vi "Main.vi"() -> ()   [LabVIEW 2014, in "SLL Tools Launcher.lvlib"]
uses:
  SLL Tools Launcher.lvlib
  Typedefs/SLL Tool.ctl
  <vilib>/Utility/error.llb/DialogType.ctl
  Source/SLL Queued State Machine/Queue Driver/Create Queue.vi
  Source/SLL Queued State Machine/Queue Driver/Enqueue an Item to Queue.vi
  Source/SLL Queued State Machine/Queue Driver/Dequeue Queue.vi
  Source/SLL Queued State Machine/Queue Driver/Enqueue N Items.vi
  Source/SLL Queued State Machine/Queue Driver/Flush Queue.vi
  Source/SLL Queued State Machine/Queue Driver/Release Queue.vi
  Source/SLL Queued State Machine/SLL QSM.lvlib
  Source/SLL File IO/SLL File IO.lvlib
panel:
  in  "SLL Tools":T1(radio)
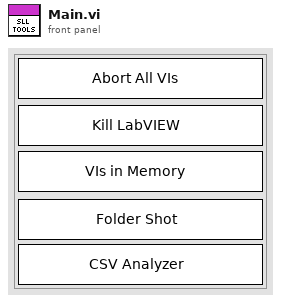
[diagram p1: front panel]
types:
  T1 = enum32{"No Selection", "Radio Selection 1", "Radio Selection 2", "Radio Selection 3", "Radio Selection 4", "Radio Selection 5"}
  T2 = typedef "SLL Tools Launcher.lvlib/SLL Tool.ctl" = cluster{"Name":string, "Path":string}
  T3 = cluster{"Flags":cluster{"Source Code?":bool}, "Selected Item":T2, "SLL Tool List[]":T2[], "Application Directory":path}
  T4 = typedef "DialogType.ctl" = u16
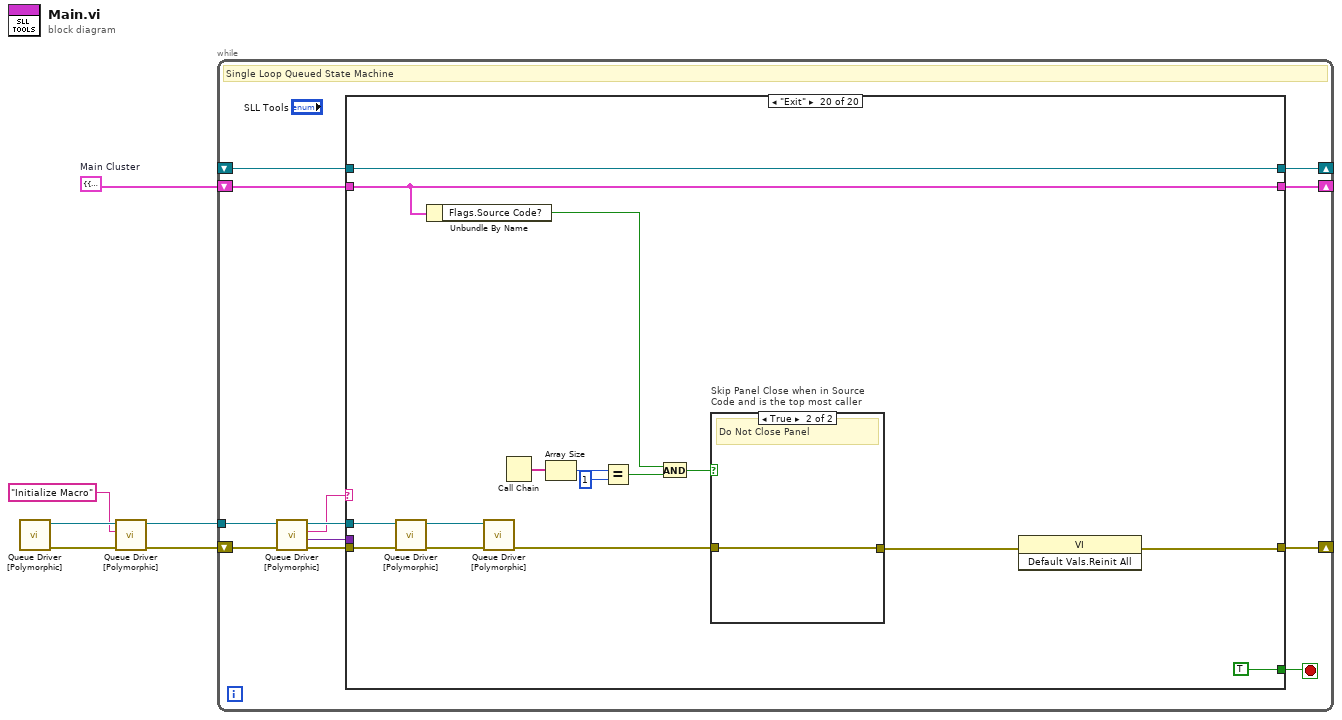
[diagram p0: block diagram]
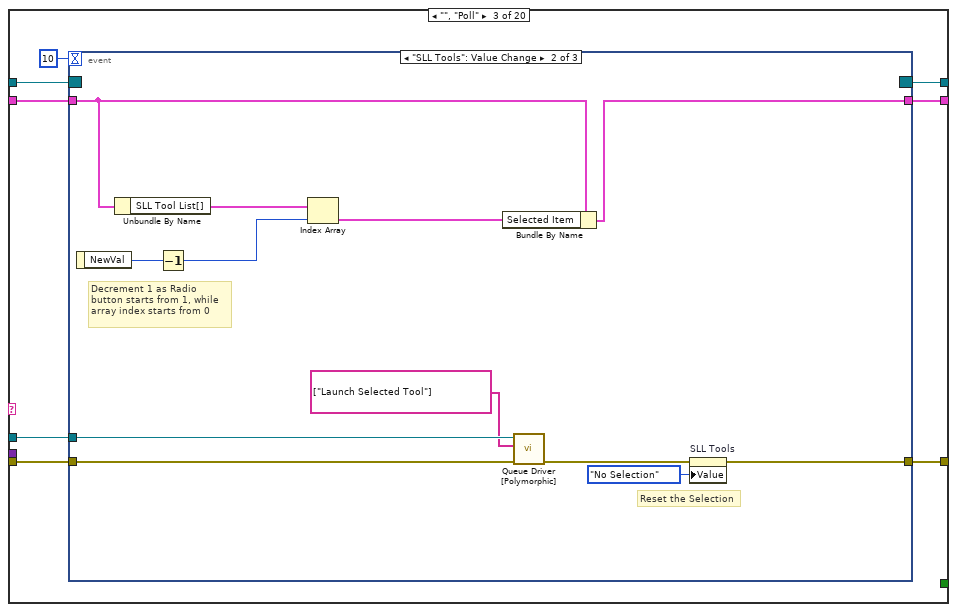
[diagram p4: hidden frame]
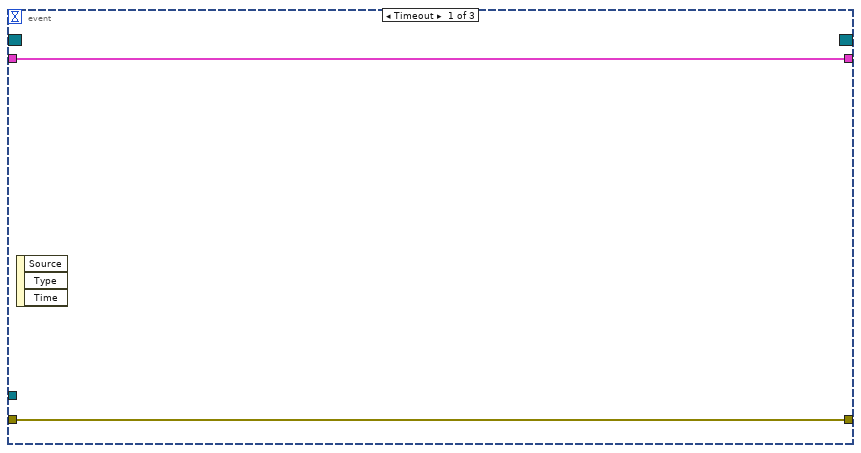
[diagram p5: hidden frame]
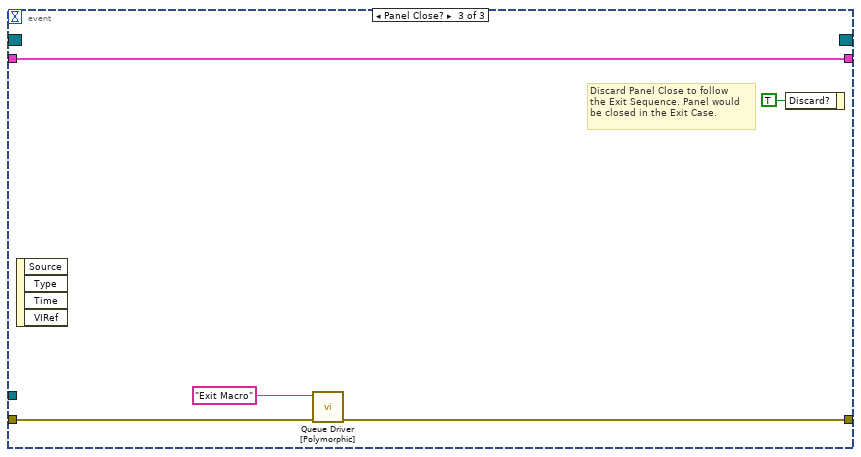
[diagram p6: hidden frame]
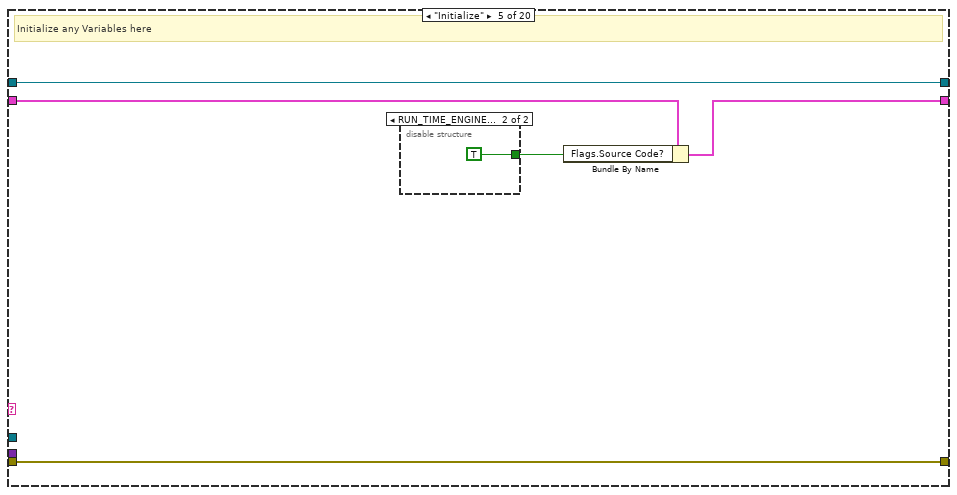
[diagram p8: hidden frame]
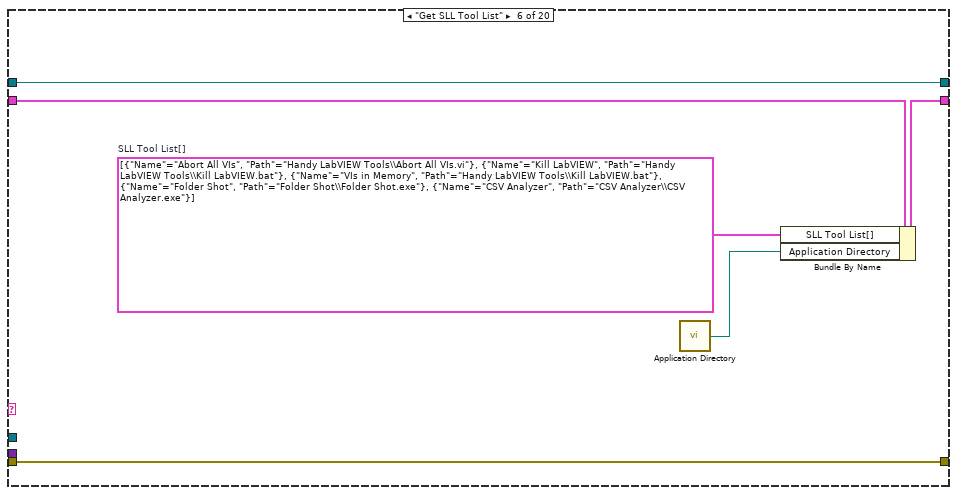
[diagram p10: hidden frame]
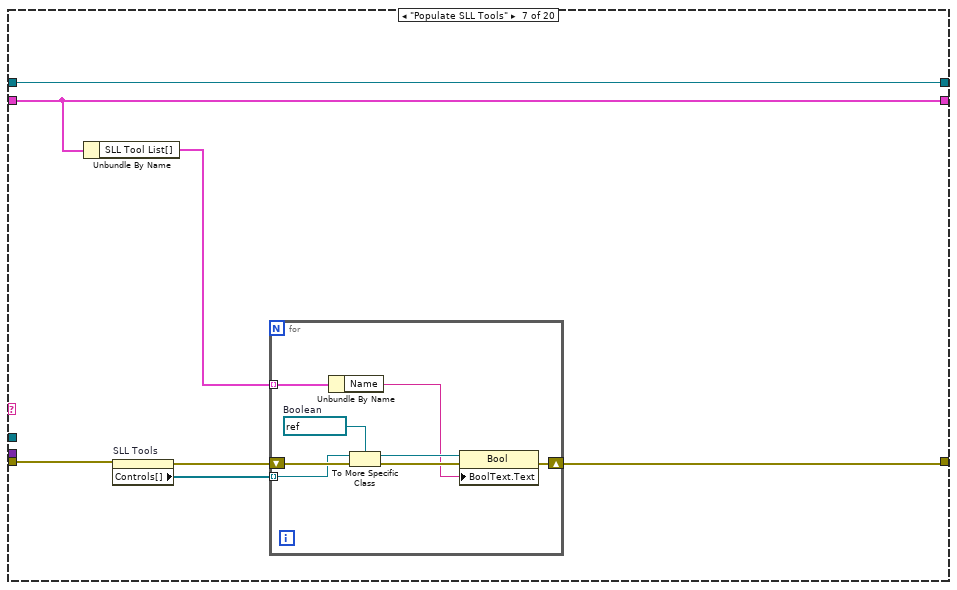
[diagram p11: hidden frame]
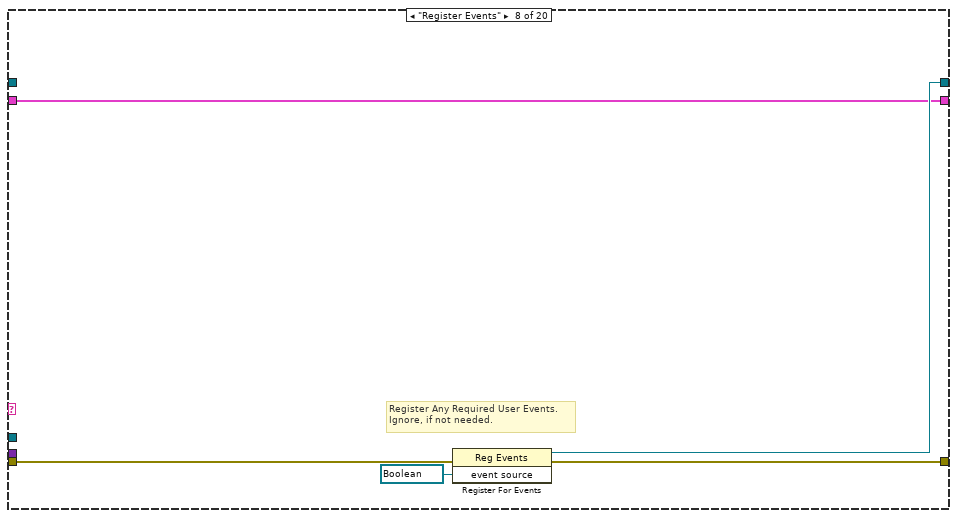
[diagram p12: hidden frame]
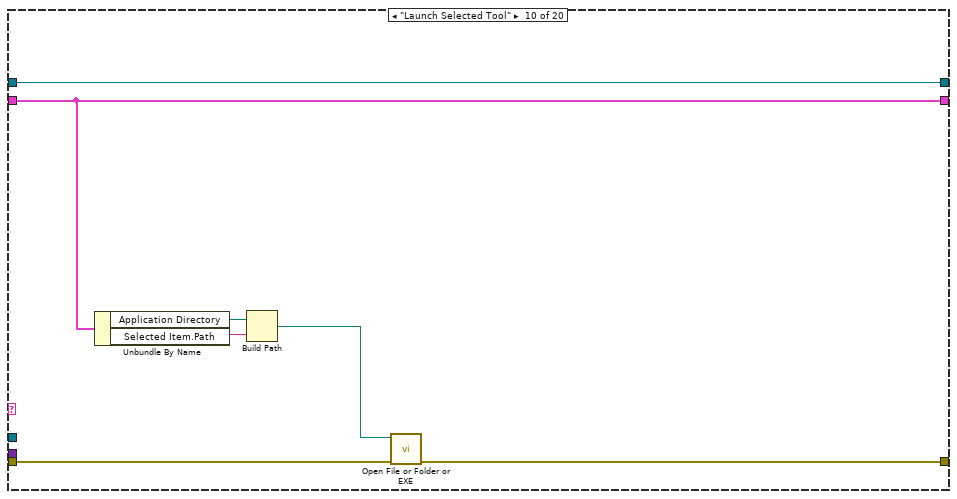
[diagram p14: hidden frame]
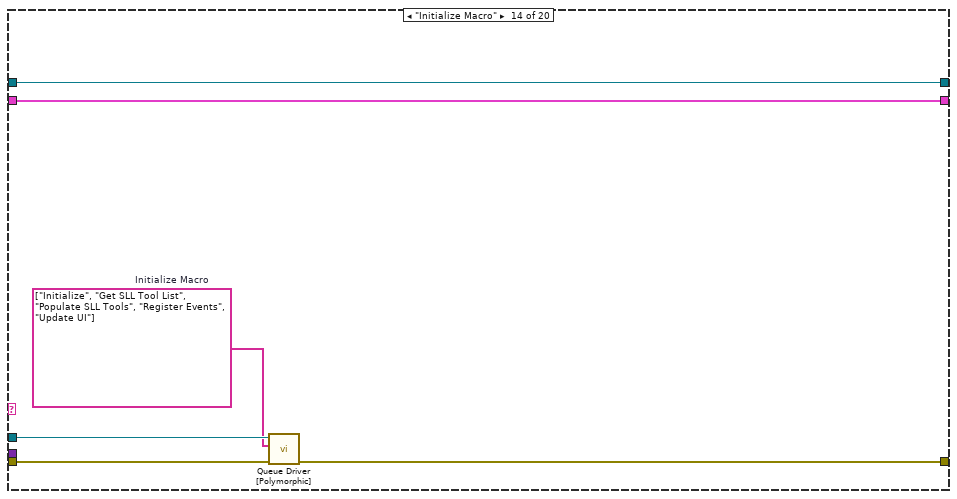
[diagram p18: hidden frame]
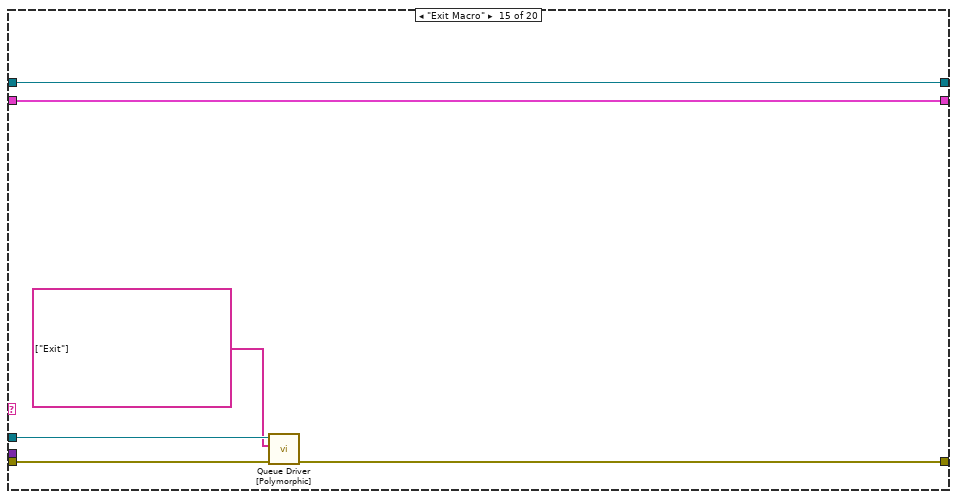
[diagram p19: hidden frame]
diagram:
  w4 = T3 {"Flags"={"Source Code?"=FALSE}, "Selected Item"={"Name"="", "Path"=""}, "SLL Tool List[]"=[], "Application Directory"=path ""}  # Main Cluster
  n1 = call-poly "Queue Driver [Polymorphic].vi"() -> ("Error Out"=w6:errorcluster, "Queue Ref"=w3:refnum<queue>)  [unwired: 10 in]
  n2 = call-poly "Queue Driver [Polymorphic].vi"("Error In"=w6, "Item to Add"="Initialize Macro", "Queue Ref In"=w3) -> ("Error Out"=w5:errorcluster, "Queue Ref Out"=w1:refnum<queue>)  [unwired: 7 in]
  n3 = while "SLL Queued State Machine" {
    shift-right: [w16] -> _
    shift-left: w5 -> [w18]
    shift-right: [w13] -> _
    shift-left: _ -> [w12]
    shift-right: [w11] -> _
    shift-left: w4 -> [w10]
    tunnel: w1 -> [w8]
    stop <- w15 stop-if-true
    # "Single Loop Queued State Machine"
    n4 = call-poly "Queue Driver [Polymorphic].vi"("Error In"=w18, "Queue Ref In"=w8) -> ("Error Out"=w17:errorcluster, "Data"=w7:variant, "Dequeue"=w9:string, "Queue Ref Out"=w14:refnum<queue>)  [unwired: 6 in]
    n5 = case "QSM Case Structure" shown="\"Exit\"" w9 {
      selector: w9 -> [_ _ _ _ _ _ _ _ _ _ _ _ _ _ _ _ w121 _ _ _]
      tunnel: w17 -> [w21 w24 w30 w54 w55 w66 w71 w86 w89 w96 w99 w102 w105 w109 w115 w120 w124 w136 w139 w153]
      tunnel: [w21 w24 w31 w54 w55 w66 w67 w85 w89 w93 w99 w102 w105 w108 w114 w120 w127 w134 w139 w142] -> w16
      tunnel: [_ _ _ _ _ _ _ _ _ _ _ _ _ _ _ _ _ _ _ TRUE] -> w15
      tunnel: [w20 w23 w29 w53 w59 w65 w73 w84 w88 w95 w98 w101 w104 w111 w117 w119 w130 w133 w138 w152] -> w13
      tunnel: w12 -> [w20 w23 w28 w53 w59 w65 w73 _ w88 w95 w98 w101 w104 w111 w117 w119 w130 w133 w138 w152]
      tunnel: [w19 w22 w26 w52 w56 w63 w72 w83 w87 w94 w97 w100 w103 w110 w116 w118 w129 w132 w137 w151] -> w11
      tunnel: w10 -> [w19 w22 w27 w52 w57 w64 w72 w83 w87 w94 w97 w100 w103 w110 w116 w118 w129 w132 w137 w151]
      tunnel: w14 -> [_ _ w25 _ _ _ _ _ _ _ _ _ _ w107 w113 _ _ _ _ w141]
      tunnel: w7 -> [_ _ _ _ _ _ _ _ _ _ _ _ _ _ _ _ _ _ _ _]
      frame "/--------------- Read Me -----------------/" {
        # "General Purpose Queue Based State Machine for Any Use Case (main application, module, pop up message etc)\n\nAdvantages:\n1. No Need to Pass Queue References between Queue Driver VIs.\n2. This template can be safely used in multiple parallel running modules without any issues.\n3. This template can also be safely used even in cases where the VI is configured to be a Clone, where multiple \ninstances of the VI could be executing concurrently.\n\nHow to Use:\n1. Add necessary items to the Main Cluster.\n2. Use the Polymorphic Queue Driver for doing any queue operations. There is no need to pass the queue driver\nreference, as the Queue Driver automatically infers the reference based on the VI instance from which it is called.\n3. Add any required user events in the \"Register Events\" case. Ignore if not needed.\n4. Use \"Sequences\" section for defining any list of state calls, which could be used in multiple places. \nEg: Initialize Sequence, might be needed if we need to any reinitialization."
      }
      frame "/------------------ Poll -------------------/" {
      }
      frame "", "Poll" {
        n6 = event shown="[1] \"SLL Tools\": Value Change" {
          selector: w28 -> [_ _ _]
          dyn-events: [_ _ _] -> w29
          timeout: 10 -> [_ _ _]
          tunnel: [w34 w38 w50] -> w31
          tunnel: w30 -> [w34 w46 w51]
          tunnel: w27 -> [w33 w45 w49]
          tunnel: [w33 w43 w49] -> w26
          tunnel: w25 -> [_ w36 _]
          event Timeout {
            n7 = event-data() -> ()  [unwired: 1 in, 3 out]
          }
          event "SLL Tools": Value Change {
            # "Reset the Selection"
            # "Decrement 1 as Radio\nbutton starts from 1, while\narray index starts from 0"
            n8 = event-data() -> ("NewVal"=w44:T1)  [unwired: 1 in]
            n9 = Unbundle By Name(w45) -> ("SLL Tool List[]"=w42:T2[])
            n10 = Decrement(x=w44) -> (x-1=w41:T1)
            n11 = Index Array(array=w42, index=w41) -> (element=w40:T2)
            n12 = Bundle By Name(cluster=w45, "Selected Item"=w40) -> (w43:T3)
            n13 = call-poly "Queue Driver [Polymorphic].vi"("Error In"=w46, "Enqueue N"=string[] ["Launch Selected Tool"], "Queue Ref In"=w36) -> ("Error Out"=w37:errorcluster)  [unwired: 7 in, 1 out]
            n14 = property on="SLL Tools" class="RadioBtnsControl (strict)"(error in=w37, "Value"=T1."No Selection" ("SLL Tools")) -> (error out=w38:errorcluster)  [unwired: 1 in, 1 out]
          }
          event Panel Close? {
            # "Discard Panel Close to follow\nthe Exit Sequence. Panel would\nbe closed in the Exit Case."
            n15 = event-data() -> ()  [unwired: 1 in, 4 out]
            n16 = call-poly "Queue Driver [Polymorphic].vi"("Error In"=w51, "Queue Name (Optional)"="Exit Macro" ("Enqueue")) -> ("Error Out"=w50:errorcluster)  [unwired: 8 in, 1 out]
            n17 = event-data("Discard?"=TRUE) -> ()  [unwired: 1 in, 1 out]
          }
        }
      }
      frame "/--------------- Initialize -----------------/" {
      }
      frame "Initialize" {
        # "Initialize any Variables here"
        n18 = disable-structure shown="RUN_TIME_ENGINE==False" {
          disable-tunnel: [_ TRUE] -> w58
          frame condition #0 {
          }
          frame condition #1 (active) {
          }
        }
        n19 = Bundle By Name(cluster=w57, "Flags.Source Code?"=w58) -> (w56:T3)
      }
      frame "Get SLL Tool List" {
        w62 = T2[] [{"Name"="Abort All VIs", "Path"="Handy LabVIEW Tools\\Abort All VIs.vi"}, {"Name"="Kill LabVIEW", "Path"="Handy LabVIEW Tools\\Kill LabVIEW.bat"}, {"Name"="VIs in Memory", "Path"="Handy LabVIEW Tools\\Kill LabVIEW.bat"}, {"Name"="Folder Shot", "Path"="Folder Shot\\Folder Shot.exe"}, {"Name"="CSV Analyzer", "Path"="CSV Analyzer\\CSV Analyzer.exe"}]  # SLL Tool List[]
        n20 = call <vilib>:"Application Directory.vi"() -> ("Application Directory"=w61:path)
        n21 = Bundle By Name(cluster=w64, "SLL Tool List[]"=w62, "Application Directory"=w61) -> (w63:T3)
      }
      frame "Populate SLL Tools" {
        n22 = Unbundle By Name(w72) -> ("SLL Tool List[]"=w68:T2[])
        n23 = property on="SLL Tools" class="RadioBtnsControl (strict)"(error in=w71) -> (error out=w70:errorcluster, "Controls[]"=w69:refnum<vi>[])  [unwired: 1 in, 1 out]
        n24 = for {
          tunnel: w69 -> [w80] mode=indexing
          shift-right: [w76] -> w67
          shift-left: w70 -> [w81]
          tunnel: w68 -> [w75] mode=indexing
          w79 = refnum<vi> refnum  # Boolean
          n25 = Unbundle By Name(w75) -> ("Name"=w74:string)
          n26 = To More Specific Class(target class=w79, reference=w80, error in=w81) -> (specific class reference=w78:refnum<vi>, error out=w77:errorcluster)
          n27 = property class="Bool"(reference=w78, error in=w77, "BoolText.Text"=w74) -> (error out=w76:errorcluster)  [unwired: 1 out]
        }
      }
      frame "Register Events" {
        # "Register Any Required User Events. \nIgnore, if not needed."
        n28 = register-events(error in=w86, refnum<vi> refnum ("event source")) -> (reference out=w84:refnum<event-registration>, error out=w85:errorcluster)  [unwired: 1 in]
      }
      frame "/---------- Functionalities ----------/" {
      }
      frame "Launch Selected Tool" {
        n29 = Unbundle By Name(w94) -> ("Application Directory"=w92:path, "Selected Item.Path"=w91:string)
        n30 = Build Path(base path=w92, name or relative path=w91) -> (appended path=w90:path)
        n31 = call "Open File or Folder or EXE.vi"("error in (no error)"=w96, "Path"=w90) -> ("error out"=w93:errorcluster)  [unwired: 9 in]
      }
      frame "/-------------- User Interface --------------/" {
        # "Duplicate this case to create additional case splitters for readability"
      }
      frame "Update UI" {
        # "Update Front Panel Controls in this Case"
      }
      frame "/----------------- Macros -----------------/" {
      }
      frame "Initialize Macro" {
        w106 = string[] ["Initialize", "Get SLL Tool List", "Populate SLL Tools", "Register Events", "Update UI"]  # Initialize Macro
        n32 = call-poly "Queue Driver [Polymorphic].vi"("Error In"=w109, "Enqueue N"=w106, "Queue Ref In"=w107) -> ("Error Out"=w108:errorcluster)  [unwired: 7 in, 1 out]
      }
      frame "Exit Macro" {
        n33 = call-poly "Queue Driver [Polymorphic].vi"("Error In"=w115, "Enqueue N"=string[] ["Exit"], "Queue Ref In"=w113) -> ("Error Out"=w114:errorcluster)  [unwired: 7 in, 1 out]
      }
      frame "/-------------- Error Handler--------------/" {
      }
      frame Default {
        # "Undefined Case/Spelling Errors - Show Message to Developer"
        n34 = property class="VI"(error in=w124) -> (error out=w123:errorcluster, "Name"=w122:string)  [unwired: 1 in, 1 out]
        n35 = Format Into String(format string="\"%s\" in the VI - %s" ("message"), initial string="Undefined case - ", error in=w123, w121, w122) -> (resulting string=w125:string, error out=w127:errorcluster)
        n36 = One Button Dialog(message=w125) -> ()  [unwired: 1 in, 1 out]
      }
      frame "Error" {
        w131 = T4 2 items=["no dialog", "OK message", "continue or stop message", "OK message + warnings", "continue/stop + warnings"] ("type of dialog (OK msg:1)")
        # "Handle the Error"
        n37 = call <vilib>:"Simple Error Handler.vi"("type of dialog (OK msg:1)"=w131, "error in (no error)"=w136) -> ("error out"=w135:errorcluster)  [unwired: 3 in, 4 out]
        n38 = call <vilib>:"Clear Errors.vi"("error in (no error)"=w135) -> ("error out"=w134:errorcluster)  [unwired: 5 in, 1 out]
      }
      frame "/------------------- Exit --------------------/" {
      }
      frame "Exit" {
        n39 = call-poly "Queue Driver [Polymorphic].vi"("Error In"=w153, "Queue Ref In"=w141) -> ("Error Out"=w154:errorcluster, "Queue Ref Out"=w140:refnum<queue>)  [unwired: 7 in, 1 out]
        n40 = Unbundle By Name(w151) -> ("Flags.Source Code?"=w144:bool)
        n41 = call-poly "Queue Driver [Polymorphic].vi"("Error In"=w154, "Queue Ref In"=w140) -> ("Error Out"=w150:errorcluster)  [unwired: 9 in]
        n42 = Call Chain() -> (call chain=w148:string[])
        n43 = Array Size(array=w148) -> (size(s)=w147:i32)
        n44 = Equal?(x=w147, y=1) -> (x = y?=w145:bool)
        n45 = And(x=w144, y=w145) -> (x .and. y?=w143:bool)
        n46 = case "Skip Panel Close when in Source\nCode and is the top most caller" shown="True" w143 {
          tunnel: w150 -> [w157 w159]
          tunnel: [w158 w159] -> w149
          frame False {
            # "Close Panel"
            n47 = invoke class="VI" method="FP.Close"() -> (error out=w156:errorcluster)  [unwired: 3 in, 2 out]
            n48 = Merge Errors(w157, w156) -> (w158:errorcluster)
          }
          frame True {
            # "Do Not Close Panel"
          }
        }
        n49 = invoke class="VI" method="Default Vals.Reinit All"(error in=w149) -> (error out=w142:errorcluster)  [unwired: 2 in, 2 out]
      }
    }
  }
